vi "sv_Get CIC Decimation Filter Coefficients.vi"(7 "reset? (True)":bool=TRUE, 8 "alias protect in final transition":bool, 9 "stop band attenuation":u16(ring) items=["72 dB", "96 dB", "120 dB"], 11 "decimation/interpolation factor":i32=16) -> (0 "delay":i32, 3 "CIC Settings":cluster{"Numeric":i32, i32, i32}, 4 "interpolation factor":i32)   [LabVIEW 2017, in "SoundVib_ContSweptSine.lvlib"]
uses:
  <vilib>/addons/Sound and Vibration/svt_Continuous Swept Sine/SoundVib_ContSweptSine.lvlib
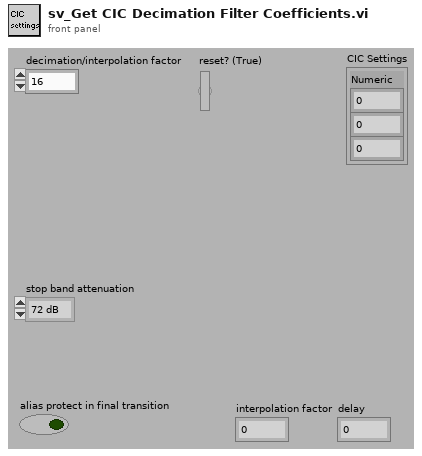
[diagram p1: front panel]
types:
  T1 = cluster{"decimation/interpolation factor":i32, i32, i32}
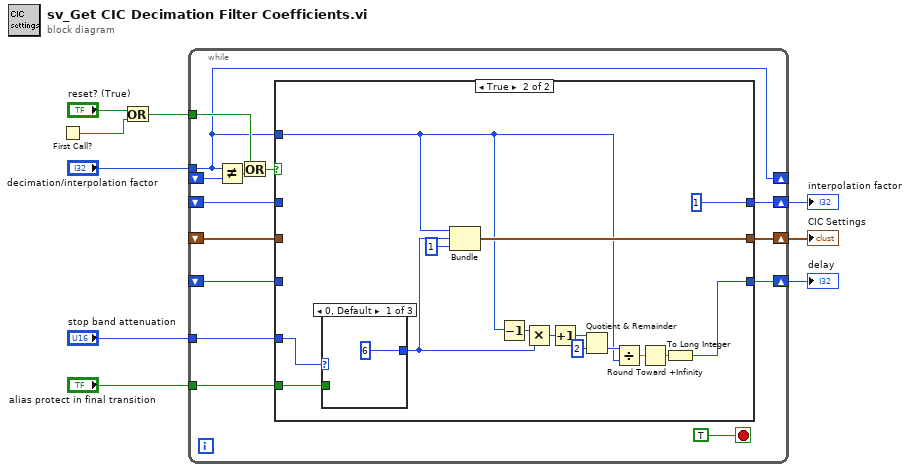
[diagram p0: block diagram]
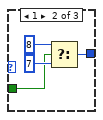
[diagram p3: hidden frame]
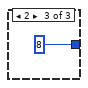
[diagram p4: hidden frame]
diagram:
  n1 = First Call?() -> (First Call?: T/F=w9:bool)
  n2 = Or(x="reset? (True)", y=w9) -> (x .or. y?=w7:bool)
  n3 = while {
    tunnel: w7 -> [w21]
    shift-right: [w12] -> _
    shift-left: _ -> [w23]
    tunnel: "decimation/interpolation factor" -> [w12]
    shift-right: [w18] -> w5
    shift-left: _ -> [w17]
    shift-right: [w16] -> w4
    shift-left: _ -> [w15]
    tunnel: "stop band attenuation" -> [w14]
    tunnel: "alias protect in final transition" -> [w13]
    shift-right: [w11] -> w1
    shift-left: _ -> [w10]
    stop <- TRUE stop-if-true
    n4 = Not Equal?(x=w12, y=w23) -> (x != y?=w22:bool)
    n5 = Or(x=w21, y=w22) -> (x .or. y?=w20:bool)
    n6 = case shown="True" w20 {
      tunnel: w12 -> [_ w28]
      tunnel: [w26 w35] -> w18
      tunnel: w17 -> [w26 _]
      tunnel: [w25 1] -> w16
      tunnel: w15 -> [w25 _]
      tunnel: w14 -> [_ w39]
      tunnel: w13 -> [_ w38]
      tunnel: [w24 w27] -> w11
      tunnel: w10 -> [w24 _]
      frame False {
      }
      frame True {
        n7 = case shown="0, Default" w39 {
          tunnel: [6 w44 8] -> w34
          tunnel: w38 -> [_ w43 _]
          frame 0, Default {
          }
          frame 1 {
            n8 = Select(t=8, s=w43, f=7) -> (s? t:f=w44:i32)
          }
          frame 2 {
          }
        }
        n9 = Bundle("decimation/interpolation factor"=w28, w34, 1) -> (w35:T1)  [unwired: 1 out]
        n10 = Decrement(x=w28) -> (x-1=w37:i32)
        n11 = Multiply(x=w37, y=w34) -> (x*y=w36:i32)
        n12 = Increment(x=w36) -> (x+1=w32:i32)
        n13 = Quotient & Remainder(x=w32, y=2) -> (floor(x/y)=w29:i32)  [unwired: 1 out]
        n14 = Divide(x=w29, y=w28) -> (x/y=w30:dbl)
        n15 = Round Toward +Infinity(x=w30) -> (ceil(x): smallest int >= x=w31:dbl)
        n16 = To Long Integer(number=w31) -> (32bit integer=w27:i32)
      }
    }
  }
  "CIC Settings" <- w5
  "interpolation factor" <- w4
  "delay" <- w1
